vi "New JSON Array (Boolean).vi"(8 "error in (no error)":errorcluster, 10 "Boolean Array":bool[](array[boolean])) -> (0 "error out":errorcluster, 3 "JSON Array out":refnum<class "JSON Array.lvclass">)   [LabVIEW 2015, in "LVJSON.lvlib" / "JSON Array.lvclass"]
uses:
  JSON Array.lvclass
  JSON Boolean/New JSON Boolean.vi
  JSON Datatype/JSON Datatype.lvclass
  JSON Boolean/JSON Boolean.lvclass
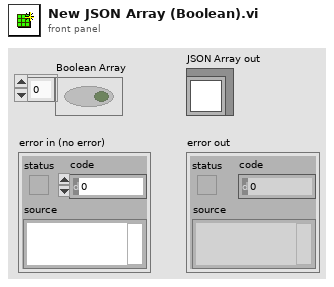
[diagram p1: front panel]
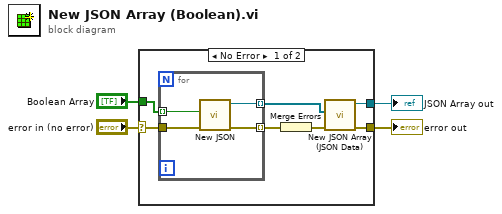
[diagram p0: block diagram]
diagram:
  n1 = case shown="No Error" "error in (no error)" {
    selector: "error in (no error)" -> [w7 w16]
    tunnel: [w9 w16] -> w3
    tunnel: [w8 _] -> w2
    tunnel: "Boolean Array" -> [w11 _]
    frame No Error {
      n2 = for {
        tunnel: w11 -> [w15] mode=indexing
        tunnel: [w14] -> w10 mode=indexing
        tunnel: w7 -> [w13]
        tunnel: [w12] -> w6 mode=indexing
        n3 = call-poly "New JSON.vi"("error in (no error)"=w13, "value"=w15) -> ("error out"=w12:errorcluster, "JSON String out"=w14:refnum<class "JSON Boolean.lvclass">)  [unwired: 8 in]
      }
      n4 = Merge Errors(w6) -> (w5:errorcluster)
      n5 = call "New JSON Array (JSON Data).vi"("error in (no error)"=w5, "JSON Datatypes"=w10) -> ("error out"=w9:errorcluster, "JSON Array out"=w8:refnum<class "JSON Array.lvclass">)  [unwired: 8 in]
    }
    frame Error {
    }
  }
  "error out" <- w3
  "JSON Array out" <- w2
